vi "19572 Get_instrument_ID.vi"(8 "error in":errorcluster, 11 "VISA resource name in":refnum<visa-resource-name>) -> (0 "error out":errorcluster, 2 "instrument ID":string, 3 "VISA resource name out":refnum<visa-resource-name>)   [LabVIEW 2015]
panel:
  # "This vi is useful in case SCPI *IDN? comand not capable to return SN number"
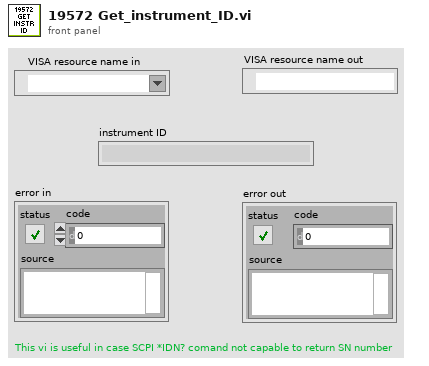
[diagram p1: front panel]
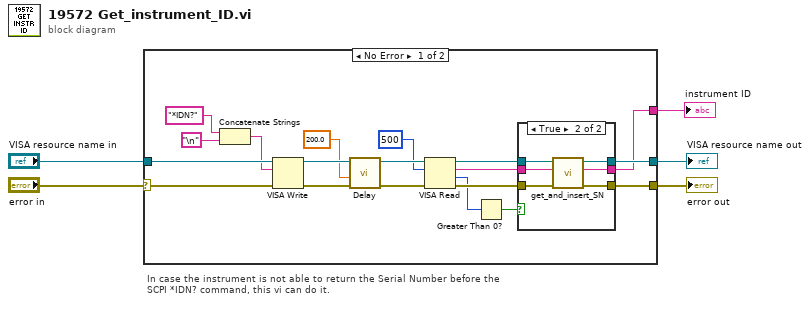
[diagram p0: block diagram]
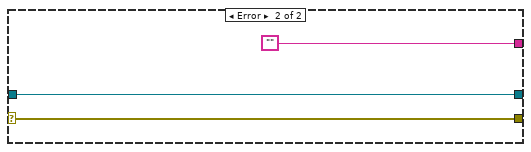
[diagram p3: hidden frame]
diagram:
  # "In case the instrument is not able to return the Serial Number before the \nSCPI *IDN? command, this vi can do it."
  n1 = case shown="No Error" "error in" {
    selector: "error in" -> [w22 w35]
    tunnel: [w14 w35] -> w5
    tunnel: [w15 w34] -> w3
    tunnel: "VISA resource name in" -> [w21 w34]
    tunnel: [w12 ""] -> w1
    frame No Error {
      n2 = Concatenate Strings("*IDN?" ("write buffer"), "\n") -> (w18:string)
      n3 = VISA Write(VISA resource name=w21, write buffer=w18, error in (no error)=w22) -> (VISA resource name out=w23:refnum<visa-resource-name>, error out=w10:errorcluster)  [unwired: 1 out]
      n4 = call "Delay.vi"("error in (no error)"=w10, "milliseconds to wait"=200.0) -> ("error out"=w9:errorcluster)  [unwired: 9 in]
      n5 = VISA Read(VISA resource name=w23, byte count=u32 500, error in (no error)=w9) -> (VISA resource name out=w16:refnum<visa-resource-name>, read buffer=w13:string, return count=w6:u32, error out=w17:errorcluster)
      n6 = Greater Than 0?(x=w6) -> (x > 0?=w7:bool)
      n7 = case shown="True" w7 {
        tunnel: w17 -> [w24 w32]
        tunnel: w16 -> [w26 w31]
        tunnel: [w26 w30] -> w15
        tunnel: [w24 w29] -> w14
        tunnel: w13 -> [w25 w28]
        tunnel: [w25 w27] -> w12
        frame False {
        }
        frame True {
          n8 = call "get_and_insert_SN.vi"("error in (no error)"=w32, "read buffer in"=w28, "VISA Refnum in"=w31) -> ("error out"=w29:errorcluster, "read buffer out"=w27:string, "VISA Refnum out"=w30:refnum<visa-resource-name>)  [unwired: 6 in]
        }
      }
    }
    frame Error {
    }
  }
  "error out" <- w5
  "VISA resource name out" <- w3
  "instrument ID" <- w1
